vi "Test Parser Compatability.vi"() -> ()   [LabVIEW 2020]
uses:
  lvsrc/subVIs/typedefs/Parsed Path - Cluster.ctl
  <vilib>/Analysis/Matrix/Datatypes/RealMatrix.ctl
  lvsrc/subVIs/typedefs/Parsed Funnel - Cluster.ctl
  lvsrc/subVIs/typedefs/Parsed Rect - Cluster.ctl
  lvsrc/Classes/Parse/ParseVectorFile/ParseVectorFile.lvclass
  C:/Program Files (x86)/National Instruments/LabVIEW 2020/vi.lib/JKI/JKI SMO/SMO/SMO.lvclass
  <vilib>/Analysis/Matrix/Comparison/Equal/Equal.vi
  <vilib>/Analysis/Matrix/Comparison/Equal/Equal - RM,RM.vi
  <vilib>/Utility/AggHandler/Cls_AggHandler.xnode
  <vilib>/JKI/JKI SMO/SMO/SMO.lvclass
  <vilib>/Analysis/Matrix/NI_Matrix.lvlib
panel:
  out "Identical?":bool
  out "Image Size 2":cluster{"Width":dbl, "Height":dbl}
  out "Image Size":cluster{"Width":dbl, "Height":dbl}
  out "Parsing Data 2":T5
  out "Parsing Data":T5
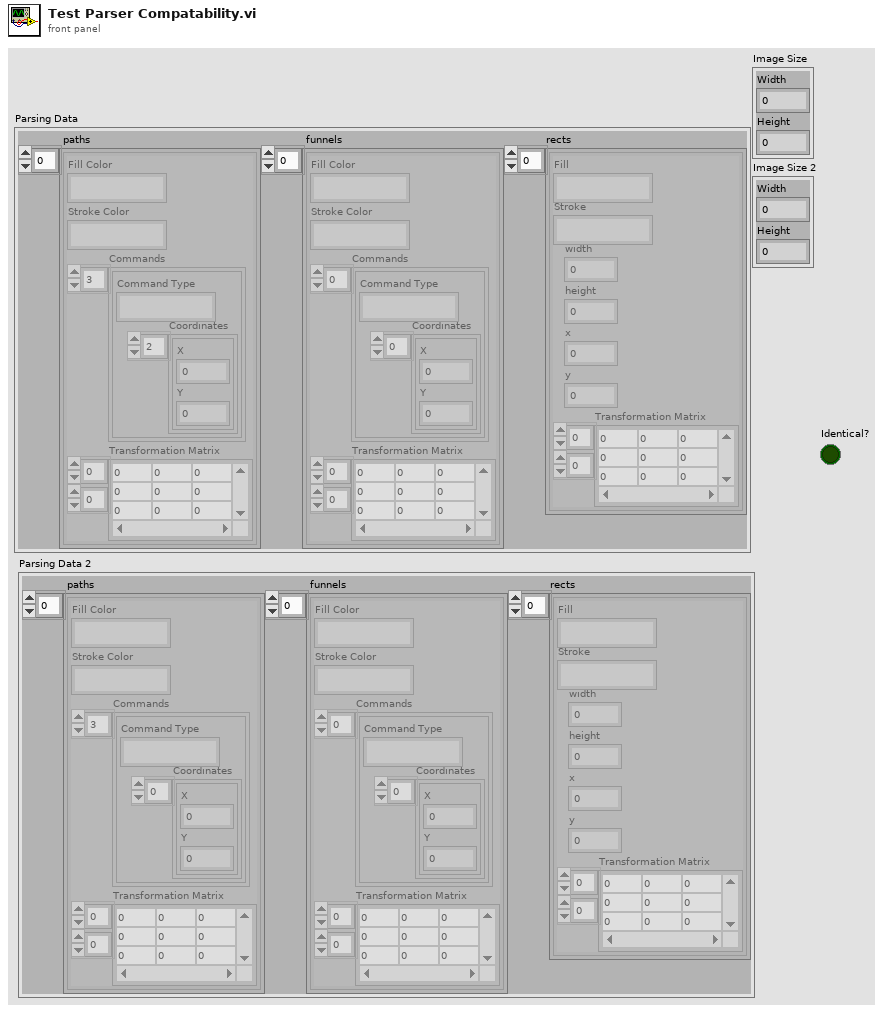
[diagram p1: front panel]
types:
  T1 = typedef "Parsed Path - Cluster.ctl" = cluster{"Fill Color":string, "Stroke Color":string, "Commands":cluster{"Command Type":string, "Coordinates":cluster{"X":dbl, "Y":dbl}[]}[], "Transformation Matrix":T2}
  T2 = typedef "NI_Matrix.lvlib/RealMatrix.ctl" = dbl[][]
  T3 = typedef "Parsed Funnel - Cluster.ctl" = cluster{"Fill Color":string, "Stroke Color":string, "Commands":cluster{"Command Type":string, "Coordinates":cluster{"X":dbl, "Y":dbl}[]}[], "Transformation Matrix":T2}
  T4 = typedef "Parsed Rect - Cluster.ctl" = cluster{"Fill":string, "Stroke":string, "width":dbl, "height":dbl, "x":dbl, "y":dbl, "Transformation Matrix":T2}
  T5 = cluster{" paths":T1[], " funnels":T3[], "rects":T4[]}
  T6 = typedef "ParseVectorFile.lvclass/PublicEvents--ParseVectorFile.ParsedData.ctl" = cluster{"Paths":refnum<class "Path.lvclass">[], "Rectangles":refnum<class "Rectangle.lvclass">[], "SVGImage":refnum<class "SVGImage.lvclass">}
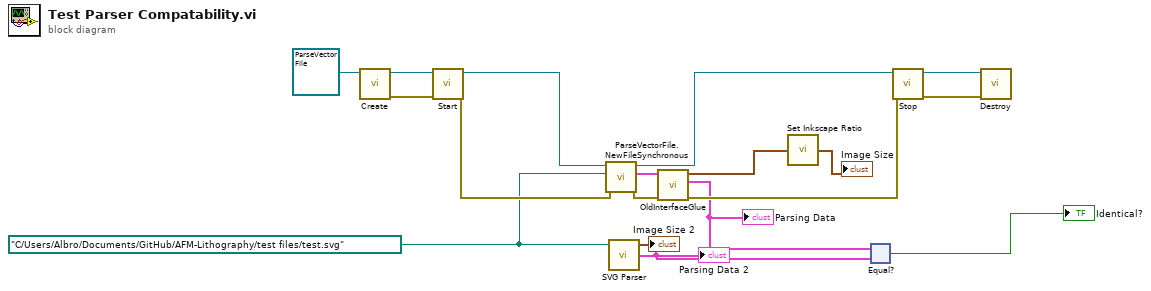
[diagram p0: block diagram]
diagram:
  w7 = path "C:/Users/Albro/Documents/GitHub/AFM-Lithography/test files/test.svg" ("XML File Path")
  n1 = call <vilib>:"Create.vi"("SMO"=refnum<class "ParseVectorFile.lvclass"> refnum ("ParseVectorFile.lvclass")) -> ("error out"=w16:errorcluster, "SMO out"=w17:refnum<class "ParseVectorFile.lvclass">)  [unwired: 8 in, 1 out]
  n2 = call <vilib>:"Start.vi"("error in (no error)"=w16, "SMO"=w17) -> ("error out"=w8:errorcluster, "SMO out"=w13:refnum<class "ParseVectorFile.lvclass">)  [unwired: 8 in]
  n3 = call "ParseVectorFile.NewFileSynchronous.vi"("error in (no error)"=w8, "Path"=w7, "ParseVectorFile"=w13) -> ("error out"=w10:errorcluster, "ParsedData"=w11:T6, "ParseVectorFile out"=w12:refnum<class "ParseVectorFile.lvclass">)  [unwired: 6 in]
  n4 = call "SVG Parser.vi"("XML File Path"=w7) -> ("Parsing Data"=w2:T5, "Image Size"=→"Image Size 2":cluster{"Width":dbl, "Height":dbl})  [unwired: 2 in, 1 out]
  "Parsing Data 2" <- w2
  n5 = call "OldInterfaceGlue.vi"("error in (no error)"=w10, "ParsedData"=w11) -> ("error out"=w9:errorcluster, "Parsing Data"=w3:T5, "Image Size"=w5:cluster{"Width":dbl, "Height":dbl})  [unwired: 7 in]
  "Parsing Data" <- w3
  n6 = call "Set Inkscape Ratio.vi"("Image Size In"=w5) -> ("Image Size Out"=→"Image Size":cluster{"Width":dbl, "Height":dbl})
  n7 = xnode "Equal?"("Y"=w2, "X"=w3) -> ("Z"=→"Identical?":bool)
  n8 = call <vilib>:"Stop.vi"("error in (no error)"=w9, "SMO"=w12) -> ("error out"=w14:errorcluster, "SMO out"=w15:refnum<class "ParseVectorFile.lvclass">)  [unwired: 8 in]
  n9 = call <vilib>:"Destroy.vi"("error in (no error)"=w14, "SMO"=w15) -> ()  [unwired: 9 in, 1 out]
